vi "Normalize by Moving Max.vi"(5 "sample length":i32, 6 "Negation":bool, 7 "Value":dbl) -> (3 "Numeric":dbl)   [LabVIEW 2019]
uses:
  <vilib>/ptbypt/NI_PtbyPt.lvlib
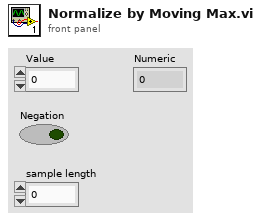
[diagram p1: front panel]
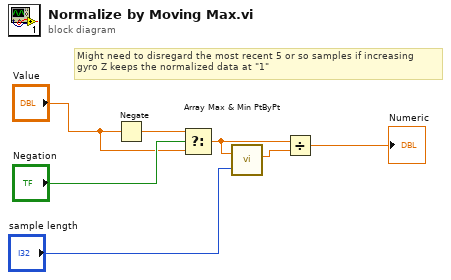
[diagram p0: block diagram]
diagram:
  # "Might need to disregard the most recent 5 or so samples if increasing\ngyro Z keeps the normalized data at \"1\""
  n1 = Negate(x="Value") -> (-x=w1:dbl)
  n2 = Select(t=w1, s="Negation", f="Value") -> (s? t:f=w2:dbl)
  n3 = call <vilib>:"Array Max & Min PtByPt.vi"("input data point"=w2, "sample length"="sample length") -> ("max value"=w3:dbl)  [unwired: 1 in, 4 out]
  n4 = Divide(x=w2, y=w3) -> (x/y=→"Numeric":dbl)
